vi "Are Digital Waveforms Equal.vi"(1 "waveform 2":digitalwaveform(waveform), 2 "waveform":digitalwaveform(waveform)) -> (0 "waveforms equal":bool)   [LabVIEW 2010]
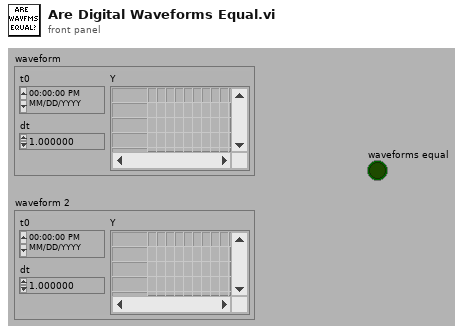
[diagram p1: front panel]
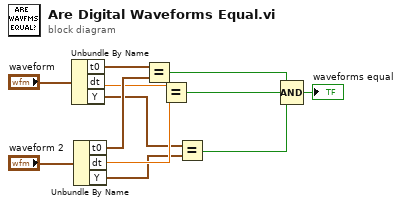
[diagram p0: block diagram]
diagram:
  n1 = Unbundle By Name("waveform") -> ("t0"=w10:timestamp, "dt"=w8:dbl, "Y"=w6:digitaldata)
  n2 = Unbundle By Name("waveform 2") -> ("t0"=w9:timestamp, "dt"=w7:dbl, "Y"=w5:digitaldata)
  n3 = Equal?(x=w10, y=w9) -> (x = y?=w4:bool)
  n4 = Equal?(x=w8, y=w7) -> (x = y?=w3:bool)
  n5 = Equal?(x=w6, y=w5) -> (x = y?=w1:bool)
  n6 = Compound Arithmetic op=AND(w4, w3, w1) -> (→"waveforms equal":bool)
